vi "LV SciSDK OSCILLOSCOPE.vi"(8 "error in (no error)":errorcluster, 9 "Oscilloscope Handle In":T2) -> (0 "error out":errorcluster, 1 "Oscilloscope Handle Out":T2, 2 "Status Code":i64, 3 "buffer out":T1)   [LabVIEW 2021]
uses:
  SciSDK_Labview.lvlib
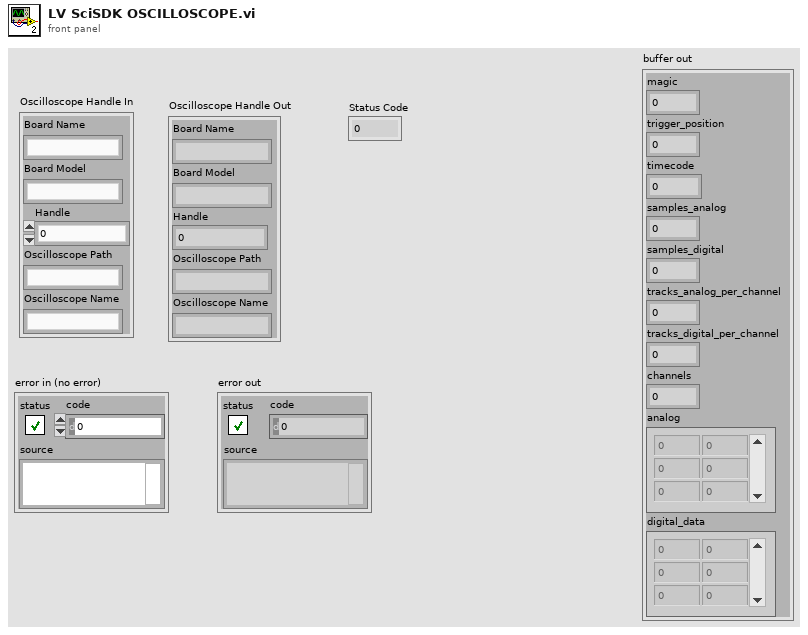
[diagram p1: front panel]
types:
  T1 = cluster{"magic":u32, "trigger_position":u64, "timecode":u64, "samples_analog":u32, "samples_digital":u32, "tracks_analog_per_channel":u32, "tracks_digital_per_channel":u32, "channels":u32, "analog":i32[][], "digital_data":i32[][]}
  T2 = cluster{"Board Name":string, "Board Model":string, "Handle":u64, "Oscilloscope Path":string, "Oscilloscope Name":string}
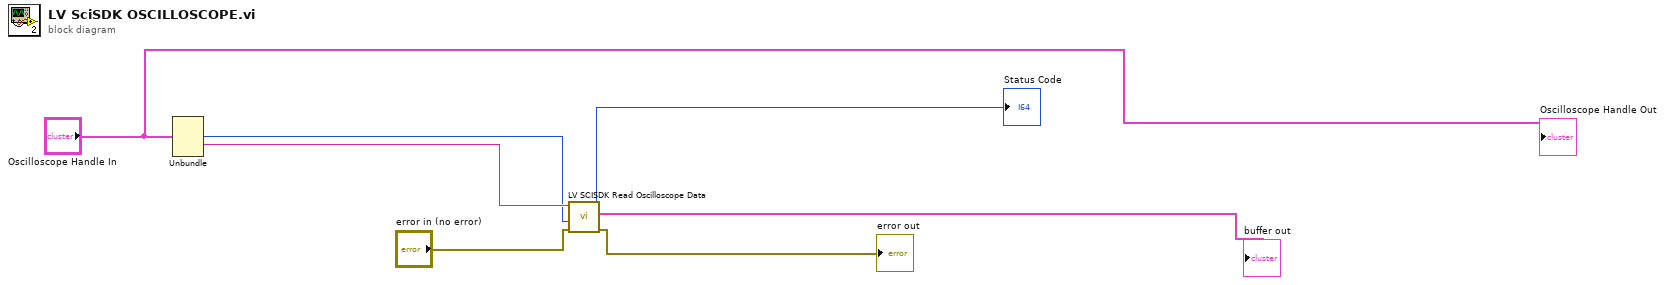
[diagram p0: block diagram]
diagram:
  n1 = Unbundle("Oscilloscope Handle In") -> ("Handle"=w6:u64, "Oscilloscope Path"=w7:string)  [unwired: 3 out]
  n2 = call "LV SCISDK Read Oscilloscope Data.vi"("Path"=w7, "handle"=w6, "error in (no error)"="error in (no error)") -> ("function return"=→"Status Code":i32, "buffer out"=→"buffer out":T1, "error out"=→"error out":errorcluster)  [unwired: 4 in, 1 out]
  "Oscilloscope Handle Out" <- "Oscilloscope Handle In"
